vi "Get API.vi"(8 "error in (no error)":errorcluster, 11 "Test 1 in":refnum<class "Test Caller.lvclass">) -> (0 "error out":errorcluster, 2 "Actor API":refnum<class "Actor API.lvclass">, 3 "Test 1 out":refnum<class "Test Caller.lvclass">)   [LabVIEW 2020, in "Scratchpad.lvlib" / "Test Caller.lvlib" / "Test Caller.lvclass"]
uses:
  Test Caller.lvclass
  Test Caller API/Test Caller API.lvclass
  Artifex/Actor Proxy/Actor API.lvclass
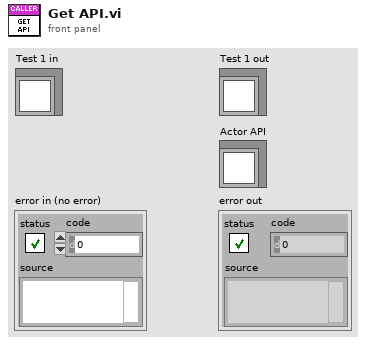
[diagram p1: front panel]
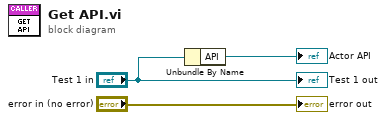
[diagram p0: block diagram]
diagram:
  n1 = Unbundle By Name("Test 1 in") -> ("API"=→"Actor API":refnum<class "Test Caller API.lvclass">)
  "error out" <- "error in (no error)"
  "Test 1 out" <- "Test 1 in"
